vi "Read Signal Samples from File and Apply Filter 2.vi"() -> ()   [LabVIEW 2014]
uses:
  <vilib>/LabVIEW Universal Transcriptor/LabVIEW to Arduino Transcriptor/Transcriptors/System API/Serial println string.vi
  <vilib>/LabVIEW Universal Transcriptor/LabVIEW to Arduino Transcriptor/Transcriptors/System API/Serial print string.vi
  <vilib>/measure/maspectr.llb/FFT Spectrum (Mag-Phase) for 1 Chan.vi
  <vilib>/LabVIEW Universal Transcriptor/LabVIEW to Arduino Transcriptor/Transcriptors/System API/Serial print frac number.vi
  <vilib>/LabVIEW Universal Transcriptor/LabVIEW Universal Transcriptor SD Card Library/File.lvclass
  <vilib>/LabVIEW Universal Transcriptor/LabVIEW Universal Transcriptor SD Card Library/LabVIEW Universal Transcriptor SD Card Library.lvlib
  <vilib>/LabVIEW Universal Transcriptor/LabVIEW to Arduino Transcriptor/Transcriptors/System API/System Serial Library Variables/System Serial Library Variables.lvlib
  <vilib>/measure/NI_MAPro.lvlib
panel:
  out "DEBUG filtered signal spectrum 2":cluster{"f0":dbl, "df":dbl, "magnitude":dbl[]}(graph)
  out "DEBUG signal output 2":sgl[](graph)
  out "DEBUG signal output":sgl[](graph)
  out "DEBUG filtered signal spectrum":cluster{"f0":dbl, "df":dbl, "magnitude":dbl[]}(graph)
  out "String Buffer":string
  out "error out":errorcluster
  in  "Error In":errorcluster
  # "DEBUG, this is part of diagram disable structure, so this will not appear in result code."
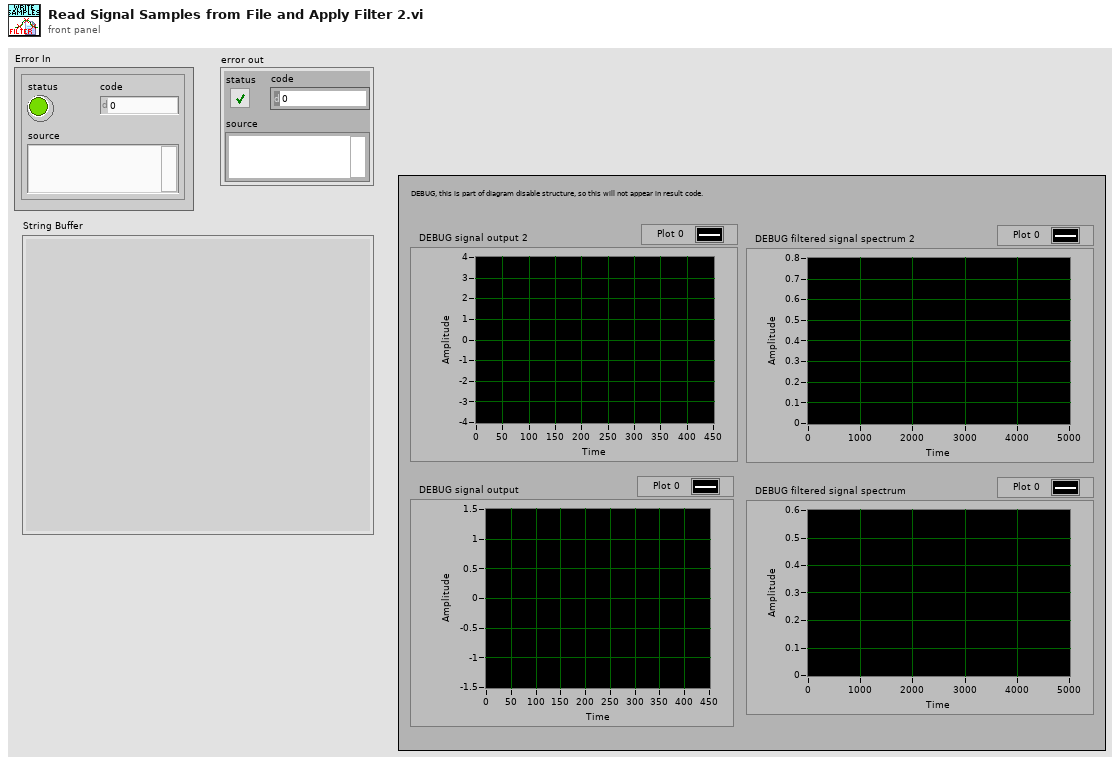
[diagram p1: front panel]
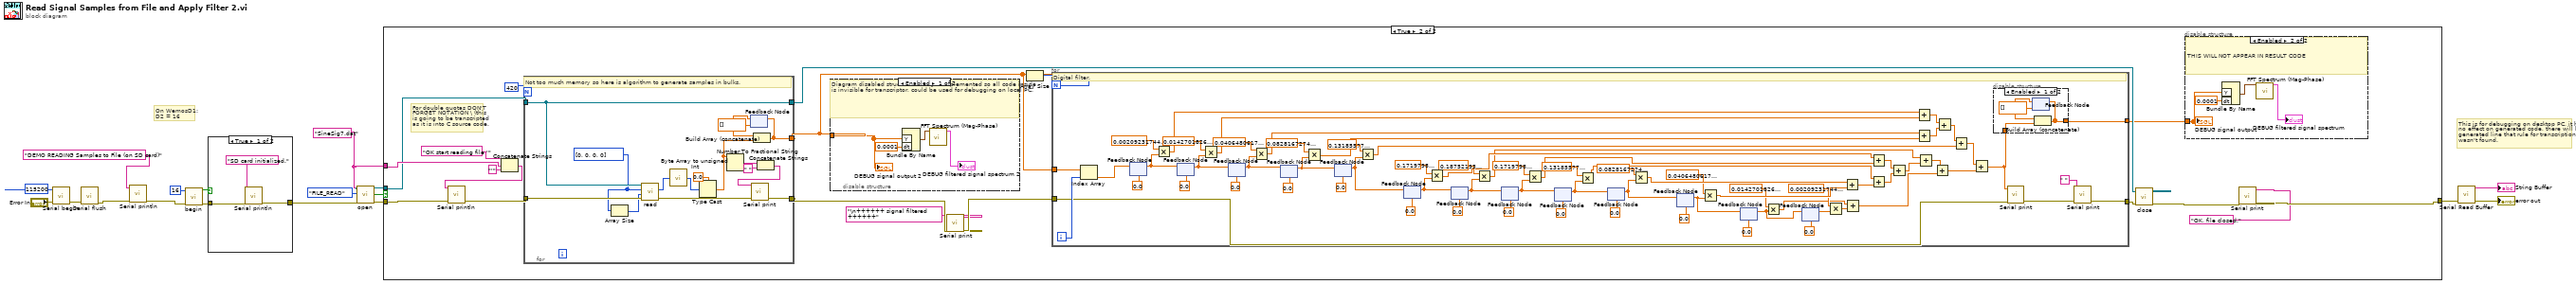
[diagram p0: block diagram]
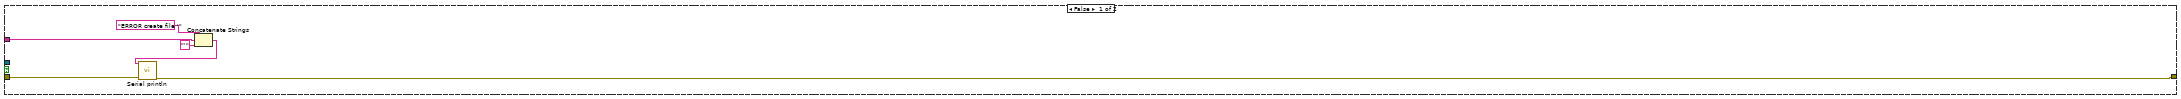
[diagram p2: hidden frame]
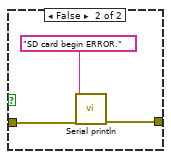
[diagram p6: hidden frame]
diagram:
  w1 = "SineSig7.dat" ("filepath")
  # "On WemosD1:\nD2 = 16"
  # "This is for debugging on desktop PC, it has\nno effect on generated code, there will be\ngenerated line that rule for transcription\nwasn't found."
  n1 = call <vilib>:"Serial begin.vi"("Error In"="Error In", "speed (Bd)"=115200) -> ("Error Out"=w18:errorcluster)  [unwired: 9 in]
  n2 = call <vilib>:"Serial flush.vi"("Error In"=w18) -> ("Error Out"=w16:errorcluster)  [unwired: 10 in]
  n3 = call-poly <vilib>:"Serial println.vi"("Error In"=w16, "string in"="DEMO READING Samples to File (on SD card)") -> ("Error Out"=w14:errorcluster)  [unwired: 9 in]
  n4 = call <vilib>:"begin.vi"("Error In"=w14, "CS pin (optional)"=u8 16) -> ("Error Out"=w11:errorcluster, "success?"=w12:bool)  [unwired: 8 in]
  n5 = case shown="True" w12 {
    tunnel: w11 -> [w21 w24]
    tunnel: [w19 w22] -> w2
    frame True {
      n6 = call-poly <vilib>:"Serial println.vi"("Error In"=w21, "string in"="SD card initialized.") -> ("Error Out"=w19:errorcluster)  [unwired: 9 in]
    }
    frame False {
      n7 = call-poly <vilib>:"Serial println.vi"("Error In"=w24, "string in"="SD card begin ERROR.") -> ("Error Out"=w22:errorcluster)  [unwired: 9 in]
    }
  }
  n8 = call <vilib>:"open.vi"("Error In"=w2, "mode"=enum16{"FILE_READ", "FILE_WRITE"}."FILE_READ", "filepath"=w1) -> ("Error Out"=w9:errorcluster, "opened?"=w8:bool, "File out"=w7:refnum<class "File.lvclass">)  [unwired: 6 in]
  n9 = case shown="True" w8 {
    tunnel: w9 -> [w26 w46]
    tunnel: w1 -> [w30 w45]
    tunnel: [w25 w35] -> w6
    tunnel: w7 -> [_ w43]
    frame False {
      n10 = Concatenate Strings("ERROR create file '" ("string in"), w30, "'" ("string")) -> (w27:string)
      n11 = call-poly <vilib>:"Serial println.vi"("Error In"=w26, "string in"=w27) -> ("Error Out"=w25:errorcluster)  [unwired: 9 in]
    }
    frame True {
      # "For double quotas DON'T\nFORGET NOTATION \\ (this\nis going to be transcripted\nas it is into C source code."
      n12 = Concatenate Strings("OK start reading file '" ("string in"), w45, "'" ("string")) -> (w47:string)
      n13 = call-poly <vilib>:"Serial println.vi"("Error In"=w46, "string in"=w47) -> ("Error Out"=w44:errorcluster)  [unwired: 9 in]
      n14 = for {
        N: 420 -> [_]
        tunnel: w44 -> [w145]
        tunnel: w43 -> [w144]
        tunnel: [w144] -> w39
        tunnel: [w149] -> w32
        tunnel: [w140] -> w40
        w143 = u8[] [0, 0, 0, 0] ("buffer")
        # "Not too much memory so here is algorithm to generate samples in bulks."
        n15 = Array Size(array=w143) -> (size(s)=w142:i32)
        n16 = call-dynamic "read.vi"("error in (no error)"=w145, "length"=w142, "buffer"=w143, "File in"=w144) -> ("error out"=w141:errorcluster, "buffer out"=w135:u8[])  [unwired: 6 in]
        n17 = call "Byte Array to unsigned Int.vi"("buffer in"=w135) -> ("unsigned int out"=w134:u32)
        n18 = Type Cast(type=sgl 0.0 ("number out"), x=w134) -> (*(type *) &x=w137:sgl)
        n19 = Number To Fractional String(number=w137) -> (F-format string=w147:string)  [unwired: 3 in]
        n20 = feedback #1(sgl[] []) -> (w138:sgl[])
        n21 = Build Array (concatenate)(w138, w137) -> (w140:sgl[])
        n22 = feedback-in #1(w140) -> ()
        n23 = Concatenate Strings(w147, " " ("element")) -> (w146:string)
        n24 = call-poly <vilib>:"Serial print.vi"("Error In"=w141, "string in"=w146) -> ("Error Out"=w149:errorcluster)  [unwired: 9 in]
      }
      n25 = disable-structure shown="Enabled" {
        disable-tunnel: w40 -> [w130 _]
        frame Enabled {
          # "Diagram disabled structure is not yet implemented so all code inside is invisible for transcriptor, could be used for debugging on local PC."
          n26 = Bundle By Name("Y"=w130, "dt"=0.0001) -> (w131:waveform(sgl))  [unwired: 1 in]
          n27 = call-poly <vilib>:"FFT Spectrum (Mag-Phase).vi"("time signal"=w131) -> ("magnitude"=→"DEBUG filtered signal spectrum 2":cluster{"f0":dbl, "df":dbl, "magnitude":dbl[]})  [unwired: 6 in, 4 out]
          "DEBUG signal output 2" <- w130
        }
        frame Disabled {
        }
      }
      n28 = call-poly <vilib>:"Serial print.vi"("Error In"=w32, "string in"="\n++++++ signal filtered ++++++") -> ("Error Out"=w33:errorcluster)  [unwired: 9 in]
      n29 = Array Size(array=w40) -> (size(s)=w41:i32)
      n30 = for {
        N: w41 -> [_]
        tunnel: w33 -> [w57]
        tunnel: w40 -> [w125]
        tunnel: [w55] -> w38
        tunnel: [w100] -> w37
        i -> [w124]
        # "Digital filter."
        n31 = Index Array(array=w125, index=w124) -> (element=w123:sgl)
        n32 = feedback-in #2(w123) -> ()
        n33 = feedback #2(sgl 0.0 ("number out")) -> (w114:sgl)
        n34 = Multiply(x=sgl 0.0020923174, y=w114) -> (x*y=w109:sgl)
        n35 = feedback #3(sgl 0.0 ("number out")) -> (w113:sgl)
        n36 = feedback-in #3(w114) -> ()
        n37 = Multiply(x=sgl 0.014270183, y=w113) -> (x*y=w108:sgl)
        n38 = feedback #4(sgl 0.0 ("number out")) -> (w112:sgl)
        n39 = feedback-in #4(w113) -> ()
        n40 = Multiply(x=sgl 0.04064806, y=w112) -> (x*y=w107:sgl)
        n41 = feedback #5(sgl 0.0 ("number out")) -> (w105:sgl)
        n42 = feedback-in #5(w112) -> ()
        n43 = Multiply(x=sgl 0.08281673, y=w105) -> (x*y=w104:sgl)
        n44 = feedback #6(sgl 0.0 ("number out")) -> (w85:sgl)
        n45 = feedback-in #6(w105) -> ()
        n46 = Multiply(x=sgl 0.13185577, y=w85) -> (x*y=w102:sgl)
        n47 = feedback #7(sgl 0.0 ("number out")) -> (w91:sgl)
        n48 = feedback-in #7(w85) -> ()
        n49 = Multiply(x=sgl 0.17197987, y=w91) -> (x*y=w81:sgl)
        n50 = feedback #8(sgl 0.0 ("number out")) -> (w90:sgl)
        n51 = feedback-in #8(w91) -> ()
        n52 = Multiply(x=sgl 0.18752193, y=w90) -> (x*y=w77:sgl)
        n53 = feedback #9(sgl 0.0 ("number out")) -> (w89:sgl)
        n54 = feedback-in #9(w90) -> ()
        n55 = Multiply(x=sgl 0.17197987, y=w89) -> (x*y=w80:sgl)
        n56 = feedback #10(sgl 0.0 ("number out")) -> (w87:sgl)
        n57 = feedback-in #10(w89) -> ()
        n58 = Multiply(x=sgl 0.13185577, y=w87) -> (x*y=w79:sgl)
        n59 = feedback #11(sgl 0.0 ("number out")) -> (w71:sgl)
        n60 = feedback-in #11(w87) -> ()
        n61 = Multiply(x=sgl 0.08281673, y=w71) -> (x*y=w75:sgl)
        n62 = feedback #12(sgl 0.0 ("number out")) -> (w63:sgl)
        n63 = feedback-in #12(w71) -> ()
        n64 = Multiply(x=sgl 0.04064806, y=w63) -> (x*y=w72:sgl)
        n65 = feedback #13(sgl 0.0 ("number out")) -> (w62:sgl)
        n66 = feedback-in #13(w63) -> ()
        n67 = Multiply(x=sgl 0.014270183, y=w62) -> (x*y=w65:sgl)
        n68 = feedback #14(sgl 0.0 ("number out")) -> (w66:sgl)
        n69 = feedback-in #14(w62) -> ()
        n70 = Multiply(x=sgl 0.0020923174, y=w66) -> (x*y=w64:sgl)
        n71 = Add(x=w75, y=w72) -> (x+y=w76:sgl)
        n72 = Add(x=w65, y=w64) -> (x+y=w59:sgl)
        n73 = Add(x=w81, y=w80) -> (x+y=w84:sgl)
        n74 = Add(x=w79, y=w76) -> (x+y=w83:sgl)
        n75 = Add(x=w84, y=w83) -> (x+y=w78:sgl)
        n76 = Add(x=w109, y=w108) -> (x+y=w110:sgl)
        n77 = Add(x=w107, y=w104) -> (x+y=w111:sgl)
        n78 = Add(x=w77, y=w78) -> (x+y=w61:sgl)
        n79 = Add(x=w61, y=w59) -> (x+y=w60:sgl)
        n80 = Add(x=w110, y=w111) -> (x+y=w103:sgl)
        n81 = Add(x=w103, y=w102) -> (x+y=w82:sgl)
        n82 = Add(x=w82, y=w60) -> (x+y=w58:sgl)
        n83 = disable-structure shown="Enabled" {
          disable-tunnel: w58 -> [w129 _]
          disable-tunnel: [w126 _] -> w100
          frame Enabled {
            n84 = feedback #15(sgl[] []) -> (w127:sgl[])
            n85 = Build Array (concatenate)(w127, w129) -> (w126:sgl[])
            n86 = feedback-in #15(w126) -> ()
          }
          frame Disabled {
          }
        }
        n87 = call-poly <vilib>:"Serial print.vi"("Error In"=w57, "number in"=w58) -> ("Error Out"=w56:errorcluster)  [unwired: 9 in]
        n88 = call-poly <vilib>:"Serial print.vi"("Error In"=w56, "string in"=" ") -> ("Error Out"=w55:errorcluster)  [unwired: 9 in]
      }
      n89 = call-dynamic "close.vi"("error in (no error)"=w38, "File in"=w39) -> ("error out"=w36:errorcluster)  [unwired: 9 in]
      n90 = disable-structure shown="Enabled" {
        disable-tunnel: w37 -> [_ w52]
        frame Disabled {
        }
        frame Enabled {
          # "THIS WILL NOT APPEAR IN RESULT CODE"
          n91 = Bundle By Name("Y"=w52, "dt"=0.0001) -> (w53:waveform(sgl))  [unwired: 1 in]
          n92 = call-poly <vilib>:"FFT Spectrum (Mag-Phase).vi"("time signal"=w53) -> ("magnitude"=→"DEBUG filtered signal spectrum":cluster{"f0":dbl, "df":dbl, "magnitude":dbl[]})  [unwired: 6 in, 4 out]
          "DEBUG signal output" <- w52
        }
      }
      n93 = call-poly <vilib>:"Serial print.vi"("Error In"=w36, "string in"="OK, file closed.") -> ("Error Out"=w35:errorcluster)  [unwired: 9 in]
    }
  }
  n94 = call <vilib>:"Serial Read Buffer.vi"("Error In"=w6) -> ("Error Out"=→"error out":errorcluster, "String Buffer"=→"String Buffer":string)  [unwired: 9 in]
